vi "StoredProcedurePlugin_Main.vi"(2 "ClassRefToActOn":refnum<vi>, 5 "error in (no error)":errorcluster, 6 "Action":T1=enum."ExecutePlugIn") -> (15 "MethodsTypes":string[](array[string]), 19 "error out":errorcluster)   [LabVIEW 2010]
uses:
  Provider_BaseClassInterface/BaseProvider_SubVIs/BaseProvider_PlugInManagerActions.ctl
panel:
  in  "_Cancel":bool
  in  "_OK":bool
  in  "InputArguements":string caption="Input argument"
  in  "StoredProcedureName":string caption="Enter the stored procedure name"
  # "This plugin creates a stored procedure VI"
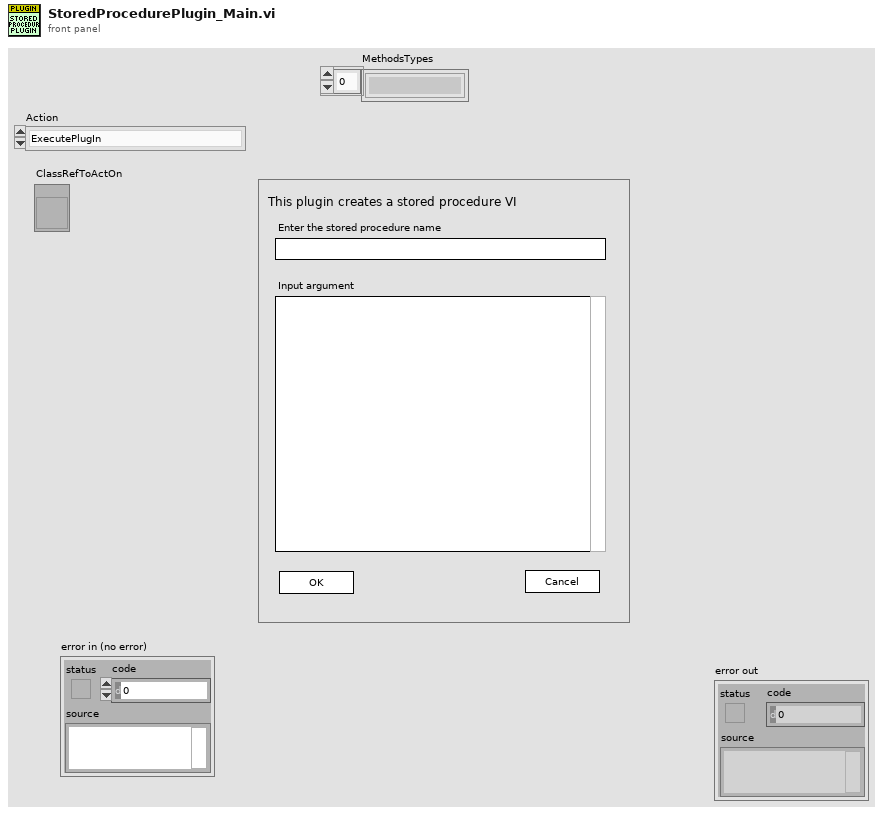
[diagram p1: front panel]
types:
  T1 = typedef "BaseProvider_PlugInManagerActions.ctl" = enum16{"GetPluginsMethods", "ExecutePlugIn"}
  T2 = cluster{"Counter":i32, "Text":string, "Cancelled":bool}
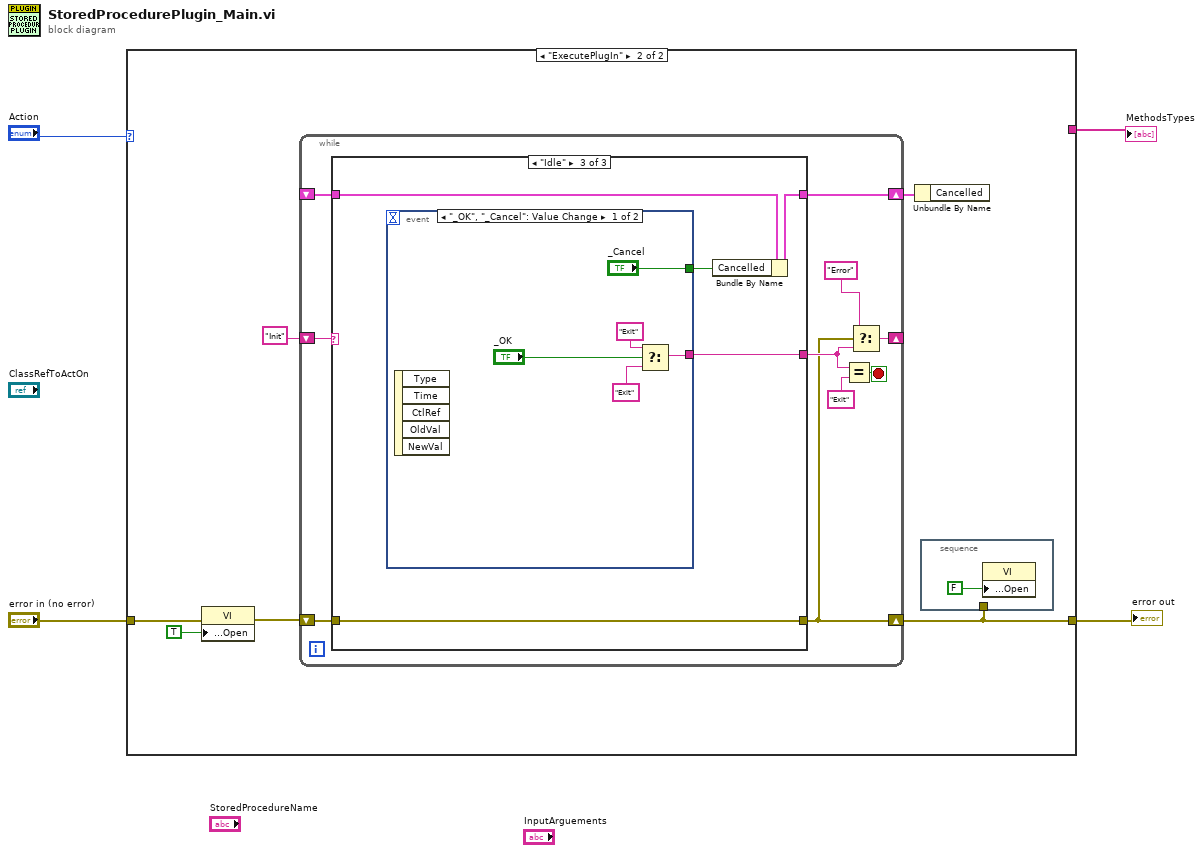
[diagram p0: block diagram]
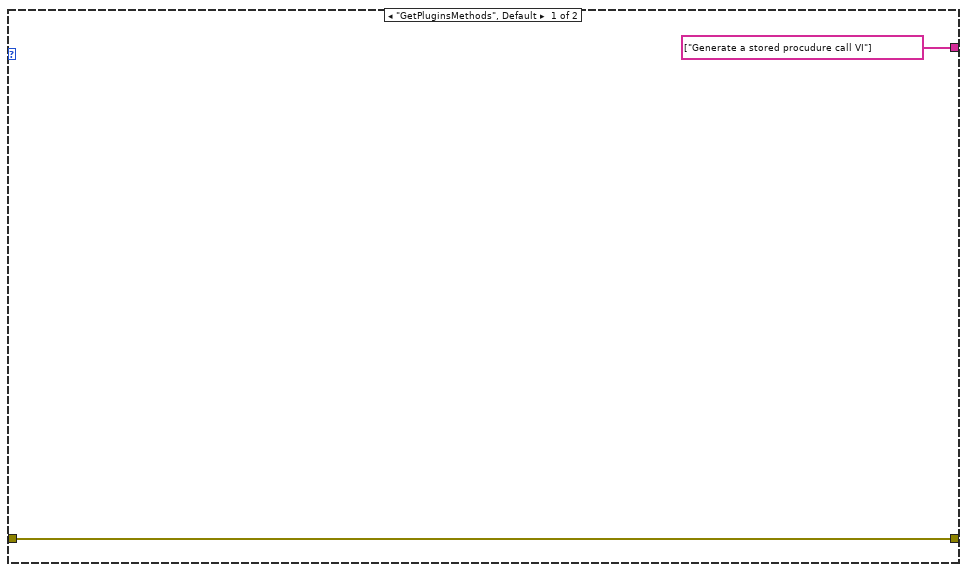
[diagram p2: hidden frame]
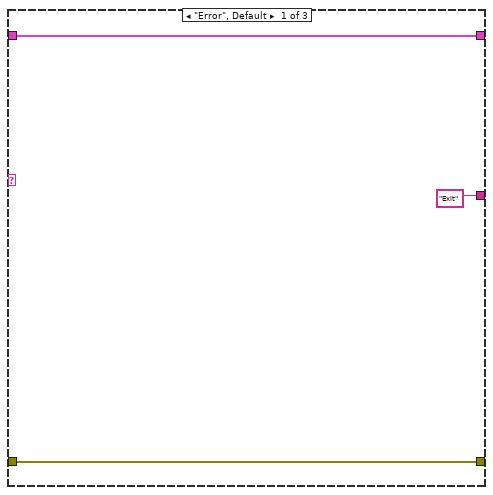
[diagram p3: hidden frame]
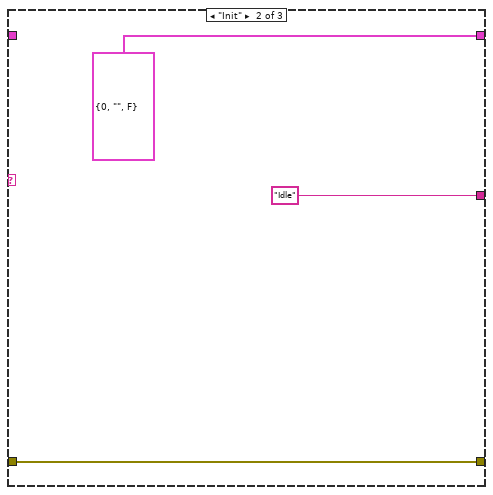
[diagram p4: hidden frame]
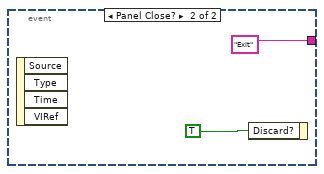
[diagram p5: hidden frame]
diagram:
  n1 = case shown="\"ExecutePlugIn\"" "Action" {
    tunnel: [string[] ["Generate a stored procudure call VI"] ("MethodsTypes") _] -> w3
    tunnel: "error in (no error)" -> [w5 w11]
    tunnel: [w5 w8] -> w1
    frame "GetPluginsMethods", Default {
    }
    frame "ExecutePlugIn" {
      n2 = property class="VI"(error in=w11, "Front Panel.Open"=TRUE ("Front Panel Window:Open")) -> (error out=w10:errorcluster)  [unwired: 1 in, 1 out]
      n3 = while {
        shift-right: [w16] -> w8
        shift-left: w10 -> [w23]
        shift-right: [w21] -> _
        shift-left: "Init" -> [w22]
        shift-right: [w15] -> w7
        shift-left: _ -> [w14]
        stop <- w20 stop-if-true
        n4 = case shown="\"Idle\"" w22 {
          tunnel: w23 -> [w26 w28 w33]
          tunnel: [w26 w28 w33] -> w16
          tunnel: ["Exit" "Idle" w34] -> w17
          tunnel: [w24 T2 {"Counter"=0, "Text"="", "Cancelled"=FALSE} w31] -> w15
          tunnel: w14 -> [w24 _ w32]
          frame "Error", Default {
          }
          frame "Init" {
          }
          frame "Idle" {
            n5 = event shown="[0] \"_OK\", \"_Cancel\": Value Change" {
              selector: _ -> [_ _]
              dyn-events: _ -> [_ _]
              timeout: _ -> [_ _]
              tunnel: [w38 "Exit"] -> w34
              tunnel: ["_Cancel" _] -> w30
              event "_OK", "_Cancel": Value Change {
                n6 = event-data() -> ()  [unwired: 1 in, 5 out]
                n7 = Select(t="Exit", s="_OK", f="Exit") -> (s? t:f=w38:string)
              }
              event Panel Close? {
                n8 = event-data() -> ()  [unwired: 1 in, 4 out]
                n9 = event-data("Discard?"=TRUE) -> ()  [unwired: 1 in, 1 out]
              }
            }
            n10 = Bundle By Name(cluster=w32, "Cancelled"=w30) -> (w31:T2)
          }
        }
        n11 = Equal?(x=w17, y="Exit") -> (x = y?=w20:bool)
        n12 = Select(t="Error", s=w16, f=w17) -> (s? t:f=w21:string)
      }
      n13 = Unbundle By Name(w7) -> ()  [unwired: 1 out]
      n14 = stacked-sequence {
        tunnel: w8 -> [_]
        frame #0 {
          n15 = property class="VI"("Front Panel.Open"=FALSE ("Front Panel Window:Open")) -> ()  [unwired: 2 in, 2 out]
        }
      }
    }
  }
  "MethodsTypes" <- w3
  "error out" <- w1
